vi "GMap Marker State Base.vi"(7 "Method":enum16{"Get", "Set"}(ring), 8 "Error In":errorcluster, 11 "Marker State In":T1) -> (0 "Error Out":errorcluster, 3 "Marker State Out":T1)   [LabVIEW 2014]
uses:
  Controls/GMap Marker State.ctl
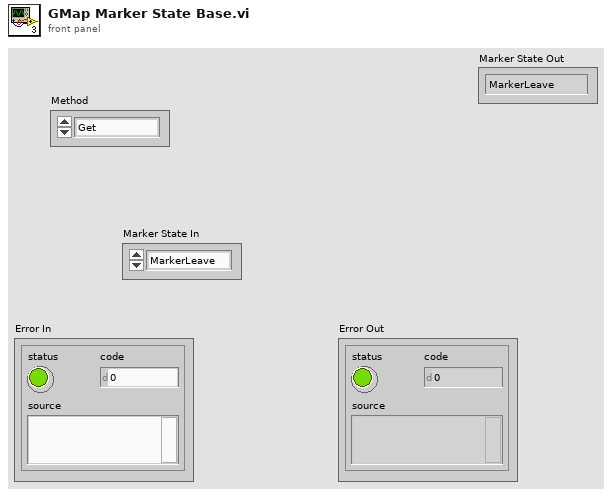
[diagram p1: front panel]
types:
  T1 = typedef "GMap Marker State.ctl" = enum16{"MarkerLeave", "MarkerEntered"}
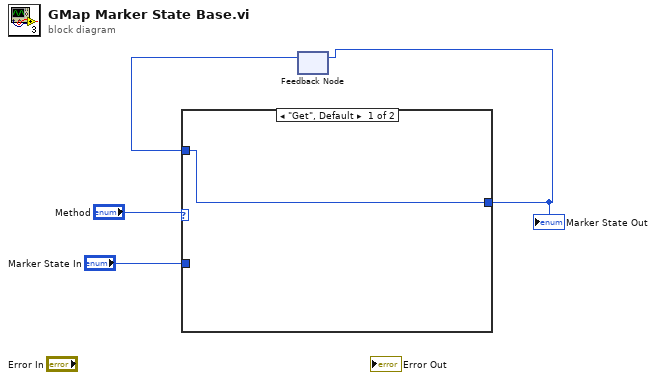
[diagram p0: block diagram]
diagram:
  n1 = feedback #1() -> (w1:T1)  [unwired: 1 in]
  n2 = case shown="\"Get\", Default" "Method" {
    tunnel: "Marker State In" -> [_ w6]
    tunnel: [w5 w6] -> w2
    tunnel: w1 -> [w5 _]
    frame "Get", Default {
    }
    frame "Set" {
    }
  }
  "Marker State Out" <- w2
  n3 = feedback-in #1(w2) -> ()
